vi "E816_Sample_Application_1.vi"() -> ()   [LabVIEW 2011]
doc: "This VI demonstrates how to initialize an E-816 system, how to move an axis and how to query for the position value of this axis.\n\nIn this example the E-816 is connected through COM port 1 with baudrate 57600. The VI runs E816_Configuration_Setup.vi with these specified settings, moves the first axis relative to its current position, waits for the movement to finish and reads the position of the axis and the error status of the controller. The diagram shows how to combine the driver VIs for these tasks. \n\nFor an example of how to command multiple axes see E816_Sample_ Application_1a.vi\n\nWarning: Before running this VI, modify the \"RS232 settings\" on the block diagram to reflect your configuration. The predefined settings provided with the VI probably do not match your system."
panel:
  in  "stop":bool
  in  "error in":errorcluster
  out "Running":bool caption="Configuration_Setup.vi is running"
  out "error out":errorcluster
  out "Position":dbl[](array[numeric]) format="%.6f"
  out "First conn. axis":string[](array[string])
  out "Identification":string
  # "This VI demonstrates how to initialize an E-816 system, how to move an axis and how to query for the position value of this axis. \nThe VI runs E816_Configuration_Setup.vi with specified settings, moves the first axis relative to its current position and reads the\nposition of this axis. The diagram shows how to combine the driver VIs for these tasks. \n\nWarning: Before running this VI, modify the interface settings on the block diagram to reflect your configuration. The predefined \n                 settings provided with the VI probably do not match your system."
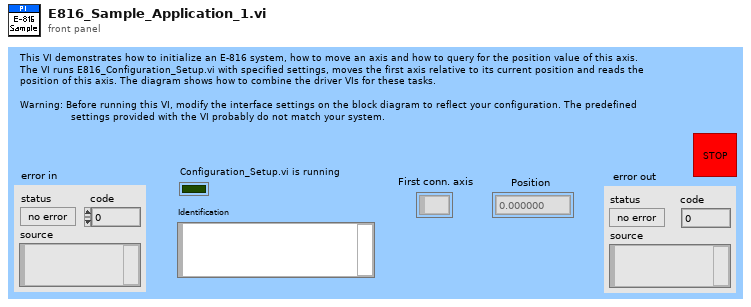
[diagram p1: front panel]
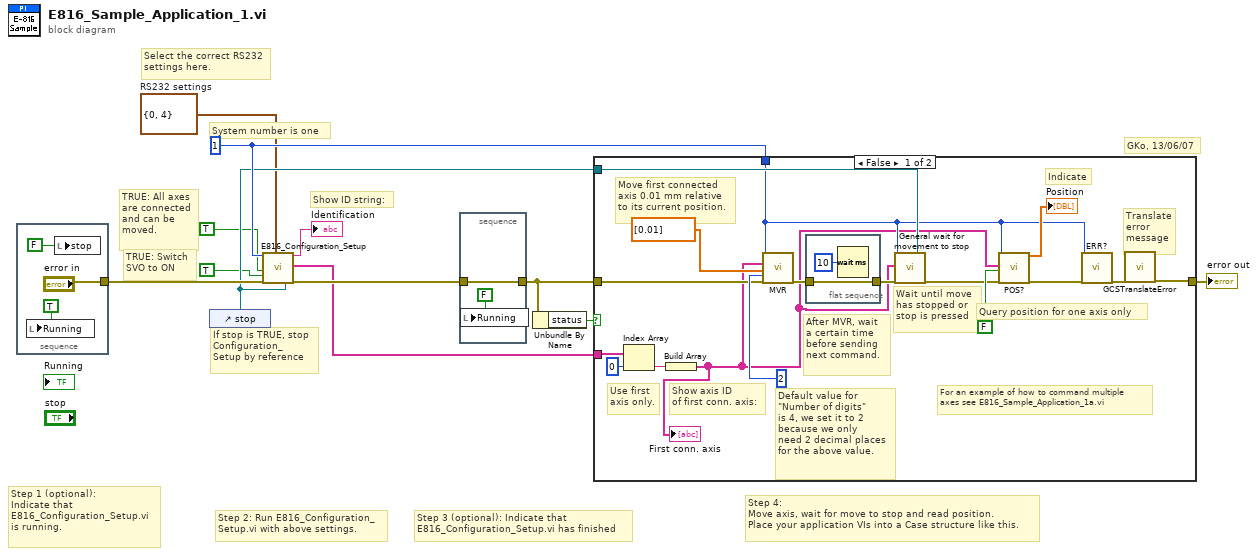
[diagram p0: block diagram]
diagram:
  w3 = cluster{"Portnumber":i32, "Baudrate":u16} {"Portnumber"=0, "Baudrate"=4}  # RS232 settings
  w8 = 1 ("System no.")
  # "TRUE: All axes\nare connected\nand can be\nmoved."
  # "TRUE: Switch\nSVO to ON"
  # "If stop is TRUE, stop\nConfiguration_\nSetup by reference"
  # "Step 4: \nMove axis, wait for move to stop and read position.\nPlace your application VIs into a Case structure like this."
  # "Select the correct RS232\nsettings here."
  # "GKo, 13/06/07"
  # "Step 3 (optional): Indicate that \nE816_Configuration_Setup.vi has finished"
  # "Step 2: Run E816_Configuration_\nSetup.vi with above settings."
  # "Step 1 (optional): \nIndicate that \nE816_Configuration_Setup.vi\nis running."
  # "Show ID string:"
  # "System number is one"
  n1 = stacked-sequence {
    tunnel: ["error in"] -> w9
    frame #0 {
      n2 = local write "Running"(TRUE ("Running")) -> ()
      n3 = local write "stop"(FALSE ("stop")) -> ()
    }
  }
  n4 = control-ref of="stop"() -> (w5:refnum<vi>)
  n5 = call "E816_Configuration_Setup.vi"("System no."=w8, "All axes?"=TRUE, "Change servo \nstatus to ON?"=TRUE ("Use dialog to define\nconnected stages?"), "error in"=w9, "RS232 settings"=w3, "Stop refnum"=w5) -> ("Identification"=→"Identification":string, "Conn. Axes"=w4:string[], "error out"=w10:errorcluster)  [unwired: 10 in, 1 out]
  n6 = stacked-sequence {
    tunnel: w10 -> [w17]
    tunnel: [w17] -> w7
    frame #0 {
      n7 = local write "Running"(FALSE ("Running")) -> ()
    }
  }
  n8 = Unbundle By Name(w7) -> ("status"=w6:bool)
  n9 = case shown="False" w6 {
    tunnel: [w29 w37] -> w11
    tunnel: w4 -> [w21 _]
    tunnel: w8 -> [w25 _]
    tunnel: w7 -> [w30 w37]
    tunnel: w5 -> [w28 _]
    frame False {
      # "Show axis ID\nof first conn. axis:"
      # "For an example of how to command multiple\naxes see E816_Sample_Application_1a.vi"
      # "Use first\naxis only."
      # "After MVR, wait\na certain time\nbefore sending\nnext command."
      # "Translate\nerror \nmessage"
      # "Wait until move\nhas stopped or\nstop is pressed"
      # "Indicate"
      # "Default value for\n\"Number of digits\"\nis 4, we set it to 2\nbecause we only\nneed 2 decimal places\nfor the above value."
      # "Move first connected\naxis 0.01 mm relative\nto its current position."
      # "Query position for one axis only"
      n10 = Index Array(array=w21, index=0) -> (element=w19:string)
      n11 = Build Array(w19) -> (w18:string[])
      "First conn. axis" <- w18
      n12 = call "MVR.vi"("System no."=w25, "Axes to move"=w18, "Position values"=dbl[] [0.01], "No.of digits"=i16 2, "error in"=w30) -> ("error out"=w23:errorcluster)  [unwired: 14 in]
      n13 = flat-sequence {
        tunnel: w23 -> [w36]
        tunnel: [w36] -> w22
        frame #0 {
          n14 = Wait (ms)(milliseconds to wait=u32 10) -> ()  [unwired: 1 out]
        }
      }
      n15 = call "General wait for movement to stop.vi"("System no."=w25, "Axes to wait for"=w18, "error in"=w22, "Stop refnum"=w28) -> ("error out"=w24:errorcluster)  [unwired: 14 in, 1 out]
      n16 = call "POS?.vi"("System no."=w25, "Axes to query"=w18, "All axes?"=FALSE, "error in"=w24) -> ("Position"=→"Position":dbl[], "error out"=w27:errorcluster)  [unwired: 14 in]
      n17 = call "ERR?.vi"("System no."=w25, "error in"=w27) -> ("error out"=w26:errorcluster)  [unwired: 16 in, 1 out]
      n18 = call "GCSTranslateError.vi"("error in"=w26) -> ("error out"=w29:errorcluster)  [unwired: 16 in, 2 out]
    }
    frame True {
      # "Error during initialization"
    }
  }
  "error out" <- w11
